vi "KB-CalOffsetAndFlatness.vi"(0 "Image In":T2(plugin-control), 1 "ROI Descriptor":T1 {"Contours"."Type" items=["No Selection", "Point", "Line", "Rectangle", "Oval", "Polygon", "Freehand Region", "Annulus", "Unused2", "Unused3", "Broken Line", "Freehand Line", "Rotated Rectangle"]}, 2 "数值 2":dbl=0.5 format="%#_13g", 3 "Row Select Laser":string(combo)="Item4", 4 "y":dbl=200.0 format="%#_13g", 5 "error in (no error)":errorcluster, 6 "Src Data":dbl[][](array[numeric])=array422x800[337600 elements], 7 "ROI  小圆":T1 {"Contours"."Type" items=["No Selection", "Point", "Line", "Rectangle", "Oval", "Polygon", "Freehand Region", "Annulus", "Unused2", "Unused3", "Broken Line", "Freehand Line", "Rotated Rectangle"]}, 9 "数值":i32) -> (12 "x-y":dbl, 13 "内外高低差-内部高到底差":dbl[](array[numeric]), 14 "外环平均高度值":dbl, 15 "子数组 2":dbl[][](array[numeric]), 16 "内环3D":dbl[][](array[numeric]), 17 "外环3D":dbl[][](array[numeric]), 19 "error Out (no error)":errorcluster)   [LabVIEW 2015]
uses:
  <vilib>/Math Plots/3D Math Plots/3D Surface/3D Surface XCtrl/3D Surface.xctl
  <vilib>/Math Plots/3D Math Plots/3D Surface/3D Surface Datatype/3D Surface Datatype.lvclass
  <vilib>/Math Plots/3D Math Plots/3D Surface/3D Surface Datatype/Public/Plot Helper (Matrix).vi
panel:
  out "3D Surface 4":refnum<class "3D Plot Datatype.lvclass">[](xcontrol) caption="内环"
  out "x/y":dbl
  out "millisecond timer value":u32
  out "3D Surface 3":refnum<class "3D Plot Datatype.lvclass">[](xcontrol) caption="三维曲面"
  out "3D Surface 2":refnum<class "3D Plot Datatype.lvclass">[](xcontrol) caption="三维曲面"
  out "x/y 2":dbl
  out "內圆平均值":dbl
  out "內圆高低差":dbl
  out "Image out Mask":T2(plugin-control)
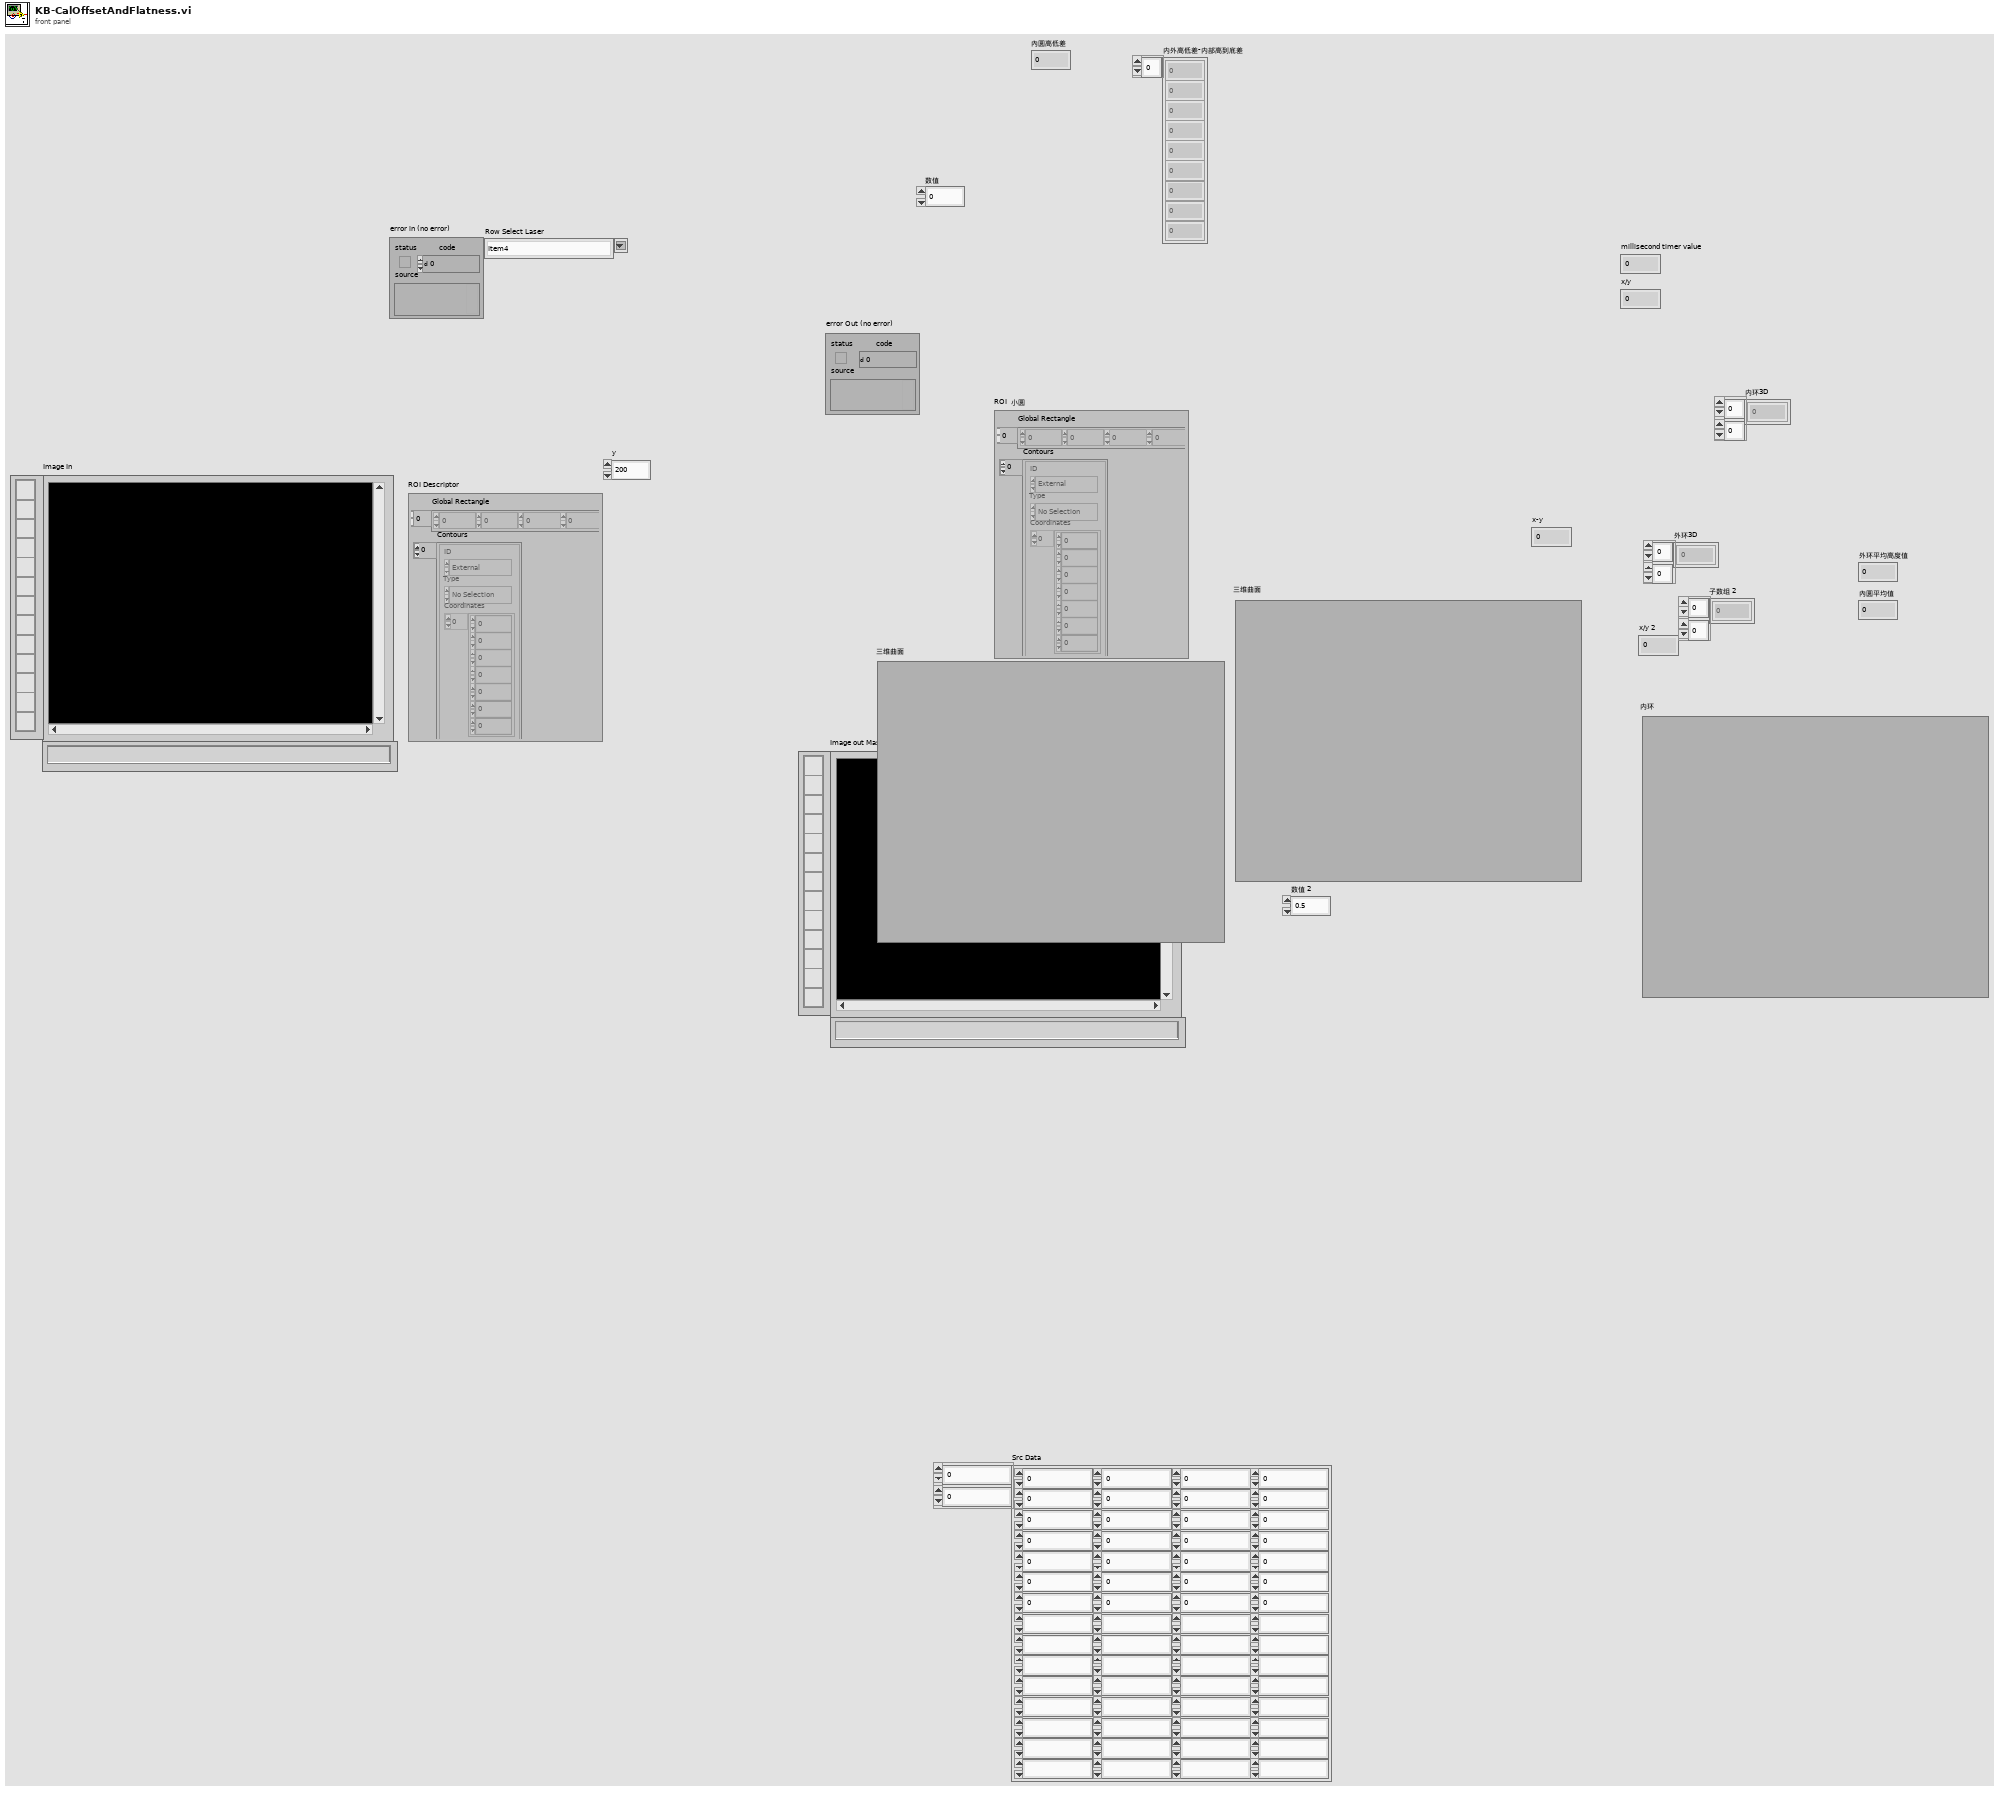
[diagram p1: front panel]
types:
  T1 = typedef "ROI Descriptor" = cluster{"Global Rectangle":i32[], "Contours":cluster{"ID":enum32{"External", "Internal"}, "Type":u32, "Coordinates":i32[]}[]}
  T2 = typedef "IMAQ Image.ctl" = refnum<image>
  T3 = cluster{"ID":enum32{"External", "Internal"}, "Type":u32, "Coordinates":i32[]}[]
  T4 = cluster{"ID":enum32{"External", "Internal"}, "Type":u32, "Coordinates":i32[]}
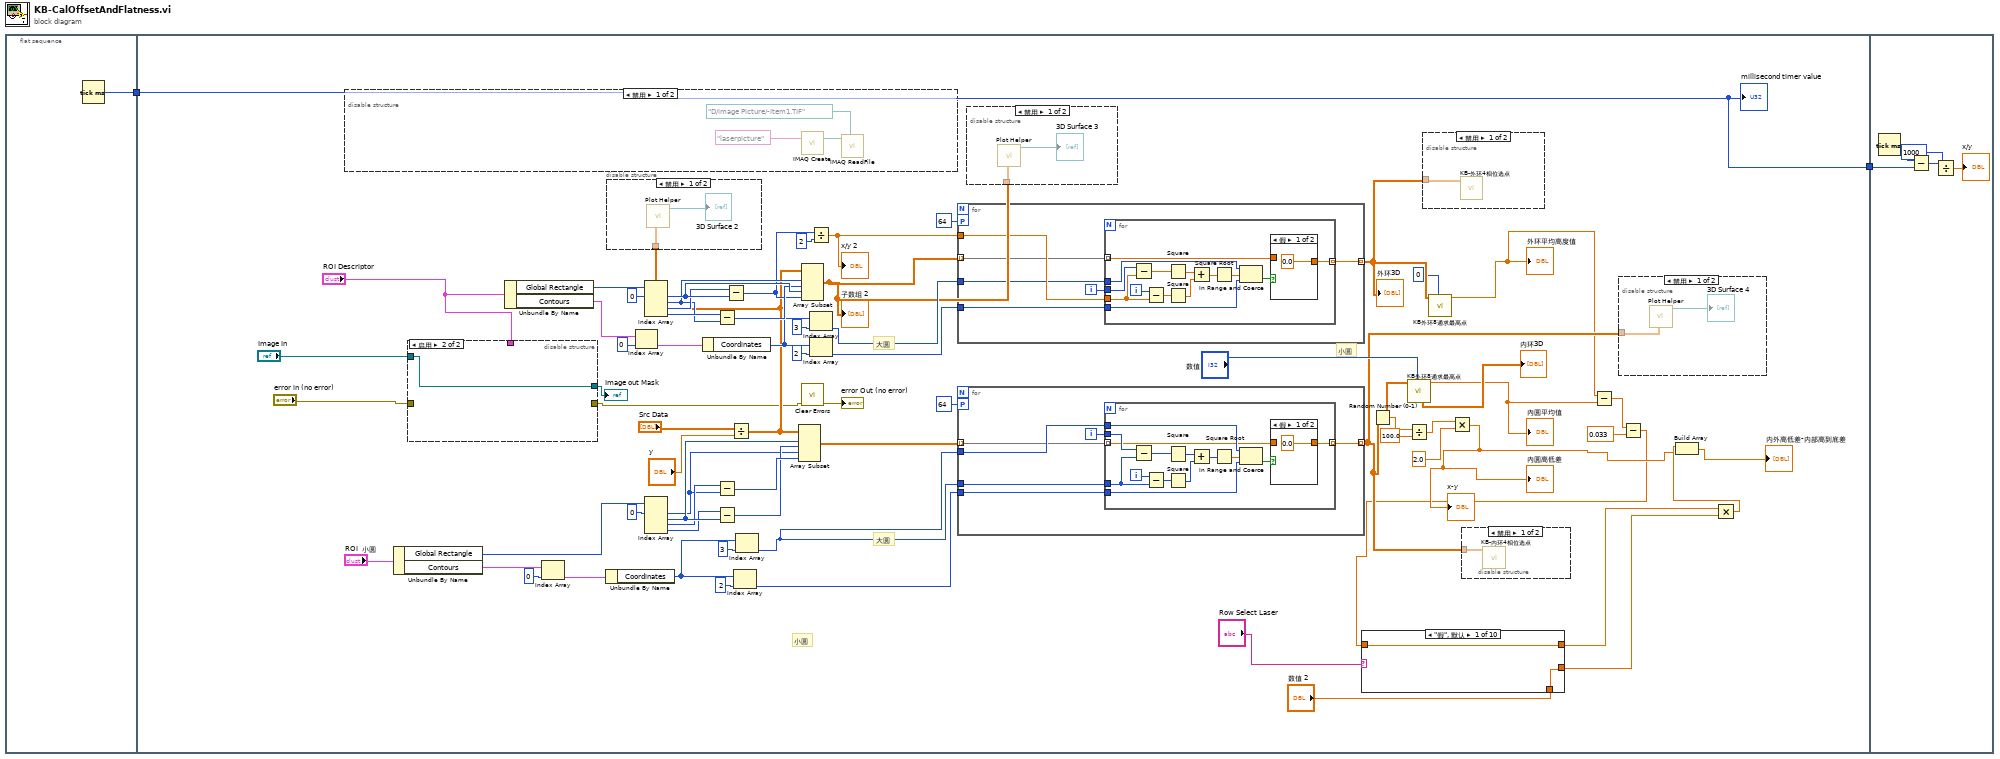
[diagram p0: block diagram]
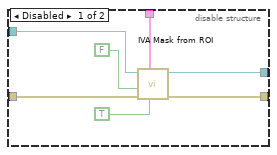
[diagram p5: hidden frame]
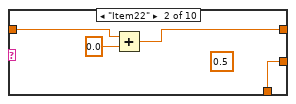
[diagram p8: hidden frame]
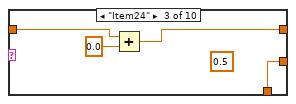
[diagram p9: hidden frame]
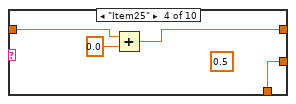
[diagram p10: hidden frame]
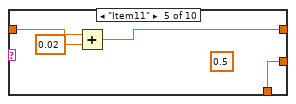
[diagram p11: hidden frame]
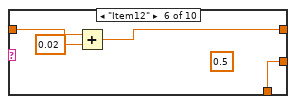
[diagram p12: hidden frame]
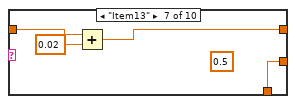
[diagram p13: hidden frame]
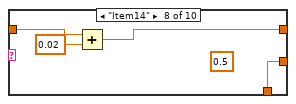
[diagram p14: hidden frame]
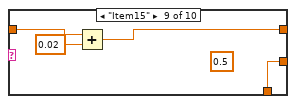
[diagram p15: hidden frame]
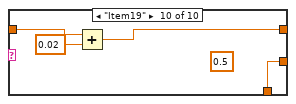
[diagram p16: hidden frame]
diagram:
  n1 = flat-sequence {
    tunnel: [w3] -> w2
    tunnel: w2 -> [w20]
    tunnel: [w20] -> w1
    tunnel: w1 -> [w178]
    frame #0 {
      n2 = Tick Count (ms)() -> (millisecond timer value=w3:u32)
    }
    frame #1 {
      # "大圆"
      # "小圆"
      # "大圆"
      # "小圆"
      n3 = disable-structure shown="禁用" {
        frame Disabled {
          n4 = call "IMAQ Create"("Image Name"="laserpicture") -> ("New Image"=w173:T2)  [unwired: 4 in, 1 out]
          n5 = call "IMAQ ReadFile"("File Path"=path "D:/image Picture/-Item1.TIF", "Image"=w173) -> ()  [unwired: 5 in, 5 out]
        }
        frame Enabled {
        }
      }
      n6 = Unbundle By Name("ROI  小圆") -> ("Global Rectangle"=w41:i32[], "Contours"=w37:T3)
      n7 = disable-structure shown="启用" {
        disable-tunnel: "error in (no error)" -> [w86 _]
        disable-tunnel: "ROI Descriptor" -> [w85 _]
        disable-tunnel: [w84 w87] -> w62
        disable-tunnel: "Image In" -> [w83 w87]
        disable-tunnel: [w80 _] -> w21
        frame Disabled {
          n8 = call <vilib>:"IVA Mask from ROI.vi"("Shrink"=TRUE, "ROI Descriptor"=w85, "error in (no error)"=w86, "Out / In"=FALSE, "Image Src"=w83) -> ("error out"=w80:errorcluster, "Image Out"=w84:T2)  [unwired: 5 out]
        }
        frame Enabled {
        }
      }
      "Image out Mask" <- w62
      n9 = Unbundle By Name("ROI Descriptor") -> ("Global Rectangle"=w69:i32[], "Contours"=w59:T3)
      n10 = Index Array(array=w37, index=0 ("索引")) -> (element=w39:T4)
      n11 = Unbundle By Name(w39) -> ("Coordinates"=w34:i32[])
      n12 = Index Array(array=w59, index=0 ("索引")) -> (element=w57:T4)
      n13 = Index Array(array=w69, index #1=0 ("索引")) -> (element #1=w67:i32, element #2=w63:i32, element #3=w65:i32, element #4=w66:i32)  [unwired: 3 in]
      n14 = Index Array(array=w41, index #1=0 ("索引")) -> (element #1=w43:i32, element #2=w47:i32, element #3=w45:i32, element #4=w44:i32)  [unwired: 3 in]
      n15 = Unbundle By Name(w57) -> ("Coordinates"=w53:i32[])
      n16 = Subtract(x=w66, y=w63) -> (x-y=w64:i32)
      n17 = Subtract(x=w45, y=w43) -> (x-y=w48:i32)
      n18 = Subtract(x=w44, y=w47) -> (x-y=w46:i32)
      n19 = Subtract(x=w65, y=w67) -> (x-y=w52:i32)
      n20 = Divide(x="Src Data", y="y") -> (x/y=w30:dbl[][])
      n21 = disable-structure shown="禁用" {
        disable-tunnel: w30 -> [w76 _]
        frame Disabled {
          n22 = call-poly <vilib>:"Plot Helper.vi"("z matrix"=w76) -> ("3D Plot lvclass Array out"=→"3D Surface 2":refnum<class "3D Plot Datatype.lvclass">[])  [unwired: 5 in, 5 out]
        }
        frame Enabled {
        }
      }
      n23 = Index Array(array=w34, index=2 ("索引")) -> (element=w33:i32)
      n24 = Index Array(array=w34, index=3 ("索引")) -> (element=w32:i32)
      n25 = Array Subset(array=w30, index (row)=w47, length (row)=w46, index (col)=w43, length (col)=w48) -> (w31:dbl[][])
      n26 = Array Subset(array=w30, index (row)=w63, length (row)=w64, index (col)=w67, length (col)=w52) -> (w29:dbl[][])
      "子数组 2" <- w29
      n27 = call <vilib>:"Clear Errors.vi"("error in (no error)"=w21) -> ("error out"=→"error Out (no error)":errorcluster)  [unwired: 5 in, 1 out]
      n28 = Divide(x=w52, y=2) -> (x/y=w50:dbl)
      "x/y 2" <- w50
      n29 = Index Array(array=w53, index=3 ("索引")) -> (element=w49:i32)
      n30 = Index Array(array=w53, index=2 ("索引")) -> (element=w55:i32)
      n31 = for {
        tunnel: w29 -> [w151] mode=indexing
        tunnel: w55 -> [w152]
        tunnel: w50 -> [w154]
        tunnel: w49 -> [w153]
        tunnel: [w150] -> w26 mode=indexing
        workers-P: 64 -> [_]
        i -> [w155]
        n32 = for {
          tunnel: w155 -> [w169]
          tunnel: w154 -> [w166]
          tunnel: w153 -> [w160]
          tunnel: w152 -> [w159]
          tunnel: w151 -> [w157] mode=indexing
          tunnel: [w156] -> w150 mode=indexing
          i -> [w167]
          n33 = Subtract(x=w169, y=w166) -> (x-y=w168:dbl)
          n34 = Subtract(x=w167, y=w166) -> (x-y=w165:dbl)
          n35 = Square(x=w168) -> (x^2=w163:dbl)
          n36 = Square(x=w165) -> (x^2=w164:dbl)
          n37 = Add(x=w163, y=w164) -> (x+y=w162:dbl)
          n38 = Square Root(x=w162) -> (sqrt(x)=w161:dbl)
          n39 = In Range and Coerce(upper limit=w160, x=w161, lower limit=w159) -> (In Range?=w158:bool)  [unwired: 1 out]
          n40 = case shown="假" w158 {
            tunnel: w157 -> [_ w171]
            tunnel: [0.0 w171] -> w156
            frame False {
            }
            frame True {
            }
          }
        }
      }
      "外环3D" <- w26
      n41 = for {
        tunnel: w31 -> [w129] mode=indexing
        tunnel: w33 -> [w130]
        tunnel: w32 -> [w132]
        tunnel: w32 -> [w131]
        tunnel: [w128] -> w15 mode=indexing
        workers-P: 64 -> [_]
        i -> [w133]
        n42 = for {
          tunnel: w133 -> [w147]
          tunnel: w132 -> [w144]
          tunnel: w131 -> [w138]
          tunnel: w130 -> [w137]
          tunnel: w129 -> [w135] mode=indexing
          tunnel: [w134] -> w128 mode=indexing
          i -> [w145]
          n43 = Subtract(x=w147, y=w144) -> (x-y=w146:i32)
          n44 = Subtract(x=w145, y=w144) -> (x-y=w143:i32)
          n45 = Square(x=w146) -> (x^2=w141:i32)
          n46 = Square(x=w143) -> (x^2=w142:i32)
          n47 = Add(x=w141, y=w142) -> (x+y=w140:i32)
          n48 = Square Root(x=w140) -> (sqrt(x)=w139:dbl)
          n49 = In Range and Coerce(upper limit=w138, x=w139, lower limit=w137) -> (In Range?=w136:bool)  [unwired: 1 out]
          n50 = case shown="假" w136 {
            tunnel: w135 -> [_ w149]
            tunnel: [0.0 w149] -> w134
            frame False {
            }
            frame True {
            }
          }
        }
      }
      n51 = disable-structure shown="禁用" {
        disable-tunnel: w29 -> [w78 _]
        frame Disabled {
          n52 = call-poly <vilib>:"Plot Helper.vi"("z matrix"=w78) -> ("3D Plot lvclass Array out"=→"3D Surface 3":refnum<class "3D Plot Datatype.lvclass">[])  [unwired: 5 in, 5 out]
        }
        frame Enabled {
        }
      }
      n53 = Random Number (0-1)() -> (number: 0 to 1=w19:dbl)
      n54 = call "KB外环8通求最高点.vi"("数值"="数值", "外环3D"=w15) -> ("平均高度"=w5:dbl, "外环3D 2"=→"内环3D":dbl[][])  [unwired: 5 in, 3 out]
      "內圆平均值" <- w5
      n55 = Divide(x=w19, y=100.0) -> (x/y=w17:dbl)
      n56 = disable-structure shown="禁用" {
        disable-tunnel: w26 -> [w89 _]
        frame Disabled {
          n57 = call "KB-外环4相位选点.vi"("外环3D"=w89) -> ()  [unwired: 8 in, 3 out]
        }
        frame Enabled {
        }
      }
      n58 = call "KB外环8通求最高点.vi"("数值"=0, "外环3D"=w26) -> ("平均高度"=w4:dbl)  [unwired: 5 in, 4 out]
      "外环平均高度值" <- w4
      n59 = Multiply(x=w17, y=2.0) -> (x*y=w8:dbl)
      "內圆高低差" <- w8
      "x-y" <- w8
      n60 = disable-structure shown="禁用" {
        disable-tunnel: w15 -> [w88 _]
        frame Disabled {
          n61 = call "KB-内环4相位选点 .vi"("内环3D"=w88) -> ()  [unwired: 7 in, 4 out]
        }
        frame Enabled {
        }
      }
      n62 = Subtract(x=w4, y=w5) -> (x-y=w10:dbl)
      n63 = disable-structure shown="禁用" {
        disable-tunnel: w15 -> [w74 _]
        frame Disabled {
          n64 = call-poly <vilib>:"Plot Helper.vi"("z matrix"=w74) -> ("3D Plot lvclass Array out"=→"3D Surface 4":refnum<class "3D Plot Datatype.lvclass">[])  [unwired: 5 in, 5 out]
        }
        frame Enabled {
        }
      }
      n65 = Subtract(x=w10, y=0.033) -> (x-y=w7:dbl)
      n66 = case shown="\"假\", 默认" "Row Select Laser" {
        tunnel: [w91 w95 w99 w103 w107 w111 w115 w119 w123 w127] -> w27
        tunnel: "数值 2" -> [w91 w95 w99 w103 w107 w111 w115 w119 w123 w127]
        tunnel: w7 -> [w90 w93 w97 w101 w105 w109 w113 w117 w121 w125]
        tunnel: [w90 w92 w96 w100 w104 w108 w112 w116 w120 w124] -> w6
        frame "假", Default {
        }
        frame "Item22" {
          (unwired) 0.5
          n67 = Add(x=w93, y=0.0) -> (x+y=w92:dbl)
        }
        frame "Item24" {
          (unwired) 0.5
          n68 = Add(x=w97, y=0.0) -> (x+y=w96:dbl)
        }
        frame "Item25" {
          (unwired) 0.5
          n69 = Add(x=w101, y=0.0) -> (x+y=w100:dbl)
        }
        frame "Item11" {
          (unwired) 0.5
          n70 = Add(x=w105, y=0.02) -> (x+y=w104:dbl)
        }
        frame "Item12" {
          (unwired) 0.5
          n71 = Add(x=w109, y=0.02) -> (x+y=w108:dbl)
        }
        frame "Item13" {
          (unwired) 0.5
          n72 = Add(x=w113, y=0.02) -> (x+y=w112:dbl)
        }
        frame "Item14" {
          (unwired) 0.5
          n73 = Add(x=w117, y=0.02) -> (x+y=w116:dbl)
        }
        frame "Item15" {
          (unwired) 0.5
          n74 = Add(x=w121, y=0.02) -> (x+y=w120:dbl)
        }
        frame "Item19" {
          (unwired) 0.5
          n75 = Add(x=w125, y=0.02) -> (x+y=w124:dbl)
        }
      }
      n76 = Multiply(x=w6, y=w27) -> (x*y=w13:dbl)
      n77 = Build Array(w13, w8) -> (→"内外高低差-内部高到底差":dbl[])
      "millisecond timer value" <- w20
    }
    frame #2 {
      n78 = Tick Count (ms)() -> (millisecond timer value=w179:u32)
      n79 = Subtract(x=w179, y=w178) -> (x-y=w177:u32)
      n80 = Divide(x=w177, y=u32 1000) -> (x/y=→"x/y":dbl)
    }
  }
